vi "Test Queues.vi"() -> ()   [LabVIEW 2020]
uses:
  Hardware/General Hardware.lvclass/General Hardware.ctl
  Hardware/Sensors/Cameras/Camera.lvclass
  C:/Users/jharw/Documents/1 Folder to Rule them All/UMD/Inflation-Apparatus/src/Hardware/General Hardware.lvclass
  Hardware/Sensors/Force Sensors/Force Sensor.lvclass
  Hardware/General Hardware.lvclass
panel:
  out "message":string
  in  "fs message":bool
  in  "cam message":bool
  in  "stop":bool
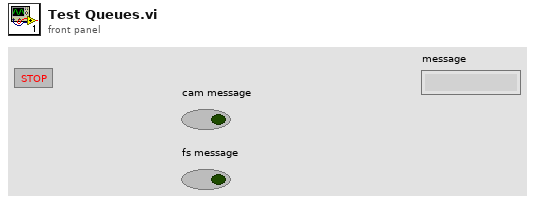
[diagram p1: front panel]
types:
  T1 = typedef "Messaging Cluster.ctl" = cluster{"cam queue":refnum<queue>, "fs queue":refnum<queue>, "servo queue":refnum<queue>, "switch queue":refnum<queue>, "cam class":refnum<class "Camera.lvclass">, "fs class":refnum<class "Force Sensor.lvclass">, "servo class":refnum<class "Servo.lvclass">, "switch class":refnum<class "Switch.lvclass">, "switch notifier":refnum<notifier>, "servo notifier":refnum<notifier>, "fs notifier":refnum<notifier>, "cam notifier":refnum<notifier>, "rgst evnt":refnum<event-registration>, "user event":refnum<user-event>, "ctlr queue":refnum<queue>}
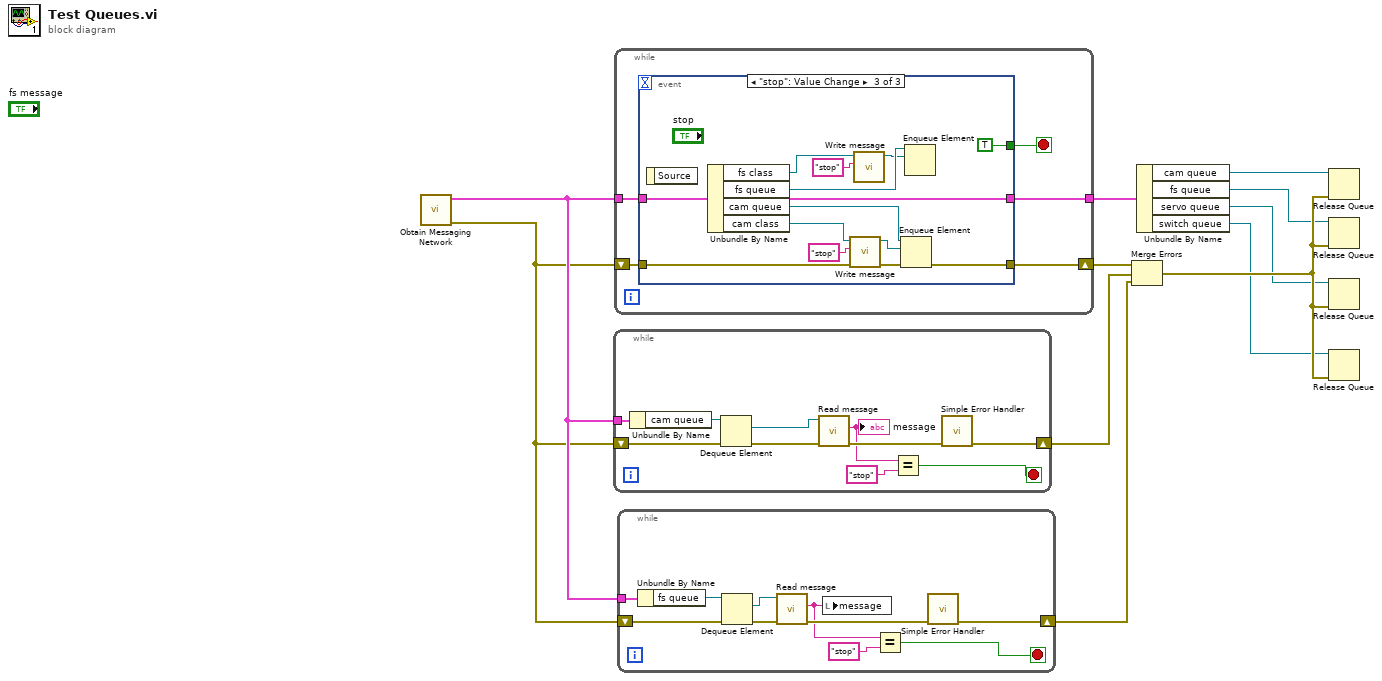
[diagram p0: block diagram]
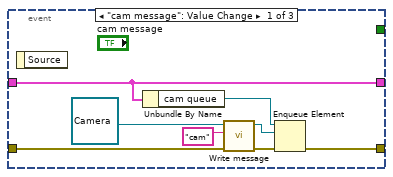
[diagram p2: hidden frame]
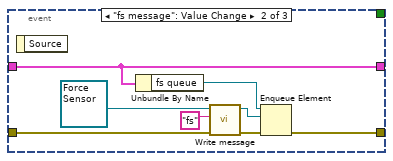
[diagram p3: hidden frame]
diagram:
  n1 = call "Obtain Messaging Network.vi"() -> ("error out"=w10:errorcluster, "msg cluster"=w11:T1)  [unwired: 10 in]
  n2 = while {
    tunnel: w11 -> [w20]
    shift-right: [w18] -> w6
    shift-left: w10 -> [w21]
    stop <- w12 stop-if-true
    n3 = Unbundle By Name(w20) -> ("cam queue"=w19:refnum<queue>)
    n4 = Dequeue Element(queue=w19, error in (no error)=w21) -> (element=w15:refnum<class "Camera.lvclass">, error out=w17:errorcluster)  [unwired: 1 in, 2 out]
    n5 = call "Read message.vi"("error in (no error)"=w17, "General Hardware in"=w15) -> ("error out"=w16:errorcluster, "message"=w14:string)  [unwired: 7 in, 1 out]
    "message" <- w14
    n6 = Equal?(x=w14, y="stop" ("message")) -> (x = y?=w12:bool)
    n7 = call <vilib>:"Simple Error Handler.vi"("error in (no error)"=w16) -> ("error out"=w18:errorcluster)  [unwired: 4 in, 4 out]
  }
  n8 = while {
    shift-right: [w24] -> w8
    shift-left: w10 -> [w26]
    tunnel: w11 -> [w25]
    tunnel: [w23] -> w9
    stop <- w22 stop-if-true
    n9 = event shown="[2] \"stop\": Value Change" {
      selector: _ -> [_ _ _]
      dyn-events: _ -> [_ _ _]
      timeout: _ -> [_ _ _]
      tunnel: w26 -> [w34 w39 w53]
      tunnel: w25 -> [w27 w35 w49]
      tunnel: [w30 w37 w51] -> w24
      tunnel: [w27 w35 w49] -> w23
      tunnel: [_ _ TRUE] -> w22
      event "cam message": Value Change {
        n10 = event-data() -> ()  [unwired: 1 in, 1 out]
        n11 = Unbundle By Name(w27) -> ("cam queue"=w28:refnum<queue>)
        n12 = call "Write message.vi"("error in (no error)"=w34, "message"="cam", "General Hardware in"=refnum<class "Camera.lvclass"> refnum ("cam class")) -> ("error out"=w33:errorcluster, "General Hardware out"=w31:refnum<class "Camera.lvclass">)  [unwired: 7 in]
        n13 = Enqueue Element(queue=w28, element=w31, error in (no error)=w33) -> (error out=w30:errorcluster)  [unwired: 1 in, 2 out]
      }
      event "fs message": Value Change {
        n14 = event-data() -> ()  [unwired: 1 in, 1 out]
        n15 = Unbundle By Name(w35) -> ("fs queue"=w40:refnum<queue>)
        n16 = call "Write message.vi"("error in (no error)"=w39, "message"="fs", "General Hardware in"=refnum<class "Force Sensor.lvclass"> refnum ("fs class")) -> ("error out"=w38:errorcluster, "General Hardware out"=w42:refnum<class "Force Sensor.lvclass">)  [unwired: 7 in]
        n17 = Enqueue Element(queue=w40, element=w42, error in (no error)=w38) -> (error out=w37:errorcluster)  [unwired: 1 in, 2 out]
      }
      event "stop": Value Change {
        n18 = event-data() -> ()  [unwired: 1 in, 1 out]
        n19 = Unbundle By Name(w49) -> ("fs class"=w46:refnum<class "Force Sensor.lvclass">, "fs queue"=w47:refnum<queue>, "cam queue"=w50:refnum<queue>, "cam class"=w44:refnum<class "Camera.lvclass">)
        n20 = call "Write message.vi"("error in (no error)"=w53, "message"="stop", "General Hardware in"=w44) -> ("error out"=w52:errorcluster, "General Hardware out"=w43:refnum<class "Camera.lvclass">)  [unwired: 7 in]
        n21 = call "Write message.vi"("message"="stop", "General Hardware in"=w46) -> ("General Hardware out"=w45:refnum<class "Force Sensor.lvclass">)  [unwired: 8 in, 1 out]
        n22 = Enqueue Element(queue=w50, element=w43, error in (no error)=w52) -> (error out=w51:errorcluster)  [unwired: 1 in, 2 out]
        n23 = Enqueue Element(queue=w47, element=w45) -> ()  [unwired: 2 in, 3 out]
      }
    }
  }
  n24 = while {
    tunnel: w11 -> [w64]
    shift-right: [w62] -> w7
    shift-left: w10 -> [w63]
    stop <- w56 stop-if-true
    n25 = Unbundle By Name(w64) -> ("fs queue"=w65:refnum<queue>)
    n26 = Dequeue Element(queue=w65, error in (no error)=w63) -> (element=w59:refnum<class "Force Sensor.lvclass">, error out=w61:errorcluster)  [unwired: 1 in, 2 out]
    n27 = call "Read message.vi"("error in (no error)"=w61, "General Hardware in"=w59) -> ("error out"=w60:errorcluster, "message"=w57:string)  [unwired: 7 in, 1 out]
    n28 = local write "message"(w57) -> ()
    n29 = Equal?(x=w57, y="stop" ("message")) -> (x = y?=w56:bool)
    n30 = call <vilib>:"Simple Error Handler.vi"("error in (no error)"=w60) -> ("error out"=w62:errorcluster)  [unwired: 4 in, 4 out]
  }
  n31 = Merge Errors(w8, w6, w7) -> (w5:errorcluster)
  n32 = Unbundle By Name(w9) -> ("cam queue"=w1:refnum<queue>, "fs queue"=w2:refnum<queue>, "servo queue"=w3:refnum<queue>, "switch queue"=w4:refnum<queue>)
  n33 = Release Queue(queue=w1, error in (no error)=w5) -> ()  [unwired: 1 in, 3 out]
  n34 = Release Queue(queue=w2, error in (no error)=w5) -> ()  [unwired: 1 in, 3 out]
  n35 = Release Queue(queue=w3, error in (no error)=w5) -> ()  [unwired: 1 in, 3 out]
  n36 = Release Queue(queue=w4, error in (no error)=w5) -> ()  [unwired: 1 in, 3 out]
